vi "OPC UA Client-Read Historical Data.vi"() -> ()   [LabVIEW 2017]
uses:
  <vilib>/OPCUA/controls/History Data.ctl
  <vilib>/OPCUA/controls/OPC UA StatusCode.ctl
  <vilib>/OPCUA/NI OPC UA Client.lvlib
panel:
  out "XY Graph":cluster{"timestamp":timestamp, dbl}[](graph)=[{"timestamp"=timestamp(3600854440.93791 s since 1904-01-01), 21.20588510972274}, {"timestamp"=timestamp(3600854441.939849 s since 1904-01-01), 27.333235009001452}, {"timestamp"=timestamp(3600854442.9396653 s since 1904-01-01), 21.855502801352223}, {"timestamp"=timestamp(3600854443.9388895 s since 1904-01-01), 29.615495560358447}, {"timestamp"=timestamp(3600854444.939037 s since 1904-01-01), 22.706889869768354}, {"timestamp"=timestamp(3600854445.940808 s since 1904-01-01), 26.35983058252613}, {"timestamp"=timestamp(3600854446.941717 s since 1904-01-01), 21.221547649340067}, {"timestamp"=timestamp(3600854447.9409194 s since 1904-01-01), 27.220020293274708}, {"timestamp"=timestamp(3600854448.94098 s since 1904-01-01), 24.57336899433289}, {"timestamp"=timestamp(3600854449.941644 s since 1904-01-01), 28.626733755791868}, {"timestamp"=timestamp(3600854450.9408674 s since 1904-01-01), 20.70668111314054}, {"timestamp"=timestamp(3600854451.9410872 s since 1904-01-01), 26.09530969102767}, {"timestamp"=timestamp(3600854452.941859 s since 1904-01-01), 29.261574143396878}, {"timestamp"=timestamp(3600854453.94282 s since 1904-01-01), 22.263766443084574}, {"timestamp"=timestamp(3600854454.9423304 s since 1904-01-01), 29.772704225559018}, {"timestamp"=timestamp(3600854455.9420905 s since 1904-01-01), 22.457297555978183}, {"timestamp"=timestamp(3600854456.942924 s since 1904-01-01), 22.19965232198119}, {"timestamp"=timestamp(3600854457.9447994 s since 1904-01-01), 21.401399761563994}, {"timestamp"=timestamp(3600854458.9439445 s since 1904-01-01), 27.088882002360943}, {"timestamp"=timestamp(3600854459.943992 s since 1904-01-01), 22.602582119449764}, {"timestamp"=timestamp(3600854460.9440994 s since 1904-01-01), 29.08142660378008}, {"timestamp"=timestamp(3600854461.9441566 s since 1904-01-01), 28.630250179567135}, {"timestamp"=timestamp(3600854462.944467 s since 1904-01-01), 21.114338923136728}, {"timestamp"=timestamp(3600854463.944479 s since 1904-01-01), 25.125580129796955}, {"timestamp"=timestamp(3600854464.9440813 s since 1904-01-01), 23.49143403146742}, {"timestamp"=timestamp(3600854465.9448175 s since 1904-01-01), 24.15475262716179}, {"timestamp"=timestamp(3600854466.944839 s since 1904-01-01), 21.48417929583267}, {"timestamp"=timestamp(3600854467.9439993 s since 1904-01-01), 27.988717224834083}, {"timestamp"=timestamp(3600854468.9438586 s since 1904-01-01), 22.36166135322488}, {"timestamp"=timestamp(3600854469.943939 s since 1904-01-01), 21.126212489266607}, {"timestamp"=timestamp(3600854470.944815 s since 1904-01-01), 23.762638809610447}, {"timestamp"=timestamp(3600854471.9439936 s since 1904-01-01), 27.854304406099796}, {"timestamp"=timestamp(3600854472.9442863 s since 1904-01-01), 20.55133627589681}, {"timestamp"=timestamp(3600854473.944202 s since 1904-01-01), 22.098002254044697}, {"timestamp"=timestamp(3600854474.9439692 s since 1904-01-01), 28.157037330075237}, {"timestamp"=timestamp(3600854475.944336 s since 1904-01-01), 27.039356091430307}, {"timestamp"=timestamp(3600854476.9447656 s since 1904-01-01), 24.751319694406348}, {"timestamp"=timestamp(3600854477.9448185 s since 1904-01-01), 23.963820168468438}, {"timestamp"=timestamp(3600854478.944527 s since 1904-01-01), 20.20490890233939}, {"timestamp"=timestamp(3600854479.944155 s since 1904-01-01), 29.410268009654118}, {"timestamp"=timestamp(3600854480.943865 s since 1904-01-01), 21.843906881862438}, {"timestamp"=timestamp(3600854481.9445095 s since 1904-01-01), 21.10194055370115}, {"timestamp"=timestamp(3600854482.9444065 s since 1904-01-01), 20.555004281742956}, {"timestamp"=timestamp(3600854483.944839 s since 1904-01-01), 28.453532206994506}, {"timestamp"=timestamp(3600854484.9440255 s since 1904-01-01), 27.422547045358044}, {"timestamp"=timestamp(3600854485.9439983 s since 1904-01-01), 20.623258344377025}, {"timestamp"=timestamp(3600854486.944007 s since 1904-01-01), 28.23587856600172}, {"timestamp"=timestamp(3600854487.9439974 s since 1904-01-01), 23.665890936914323}, {"timestamp"=timestamp(3600854488.943952 s since 1904-01-01), 29.514702727179603}, {"timestamp"=timestamp(3600854489.944659 s since 1904-01-01), 24.022882267529802}, {"timestamp"=timestamp(3600854490.9439135 s since 1904-01-01), 26.30617869644069}, {"timestamp"=timestamp(3600854491.944177 s since 1904-01-01), 24.015406120491846}, {"timestamp"=timestamp(3600854492.944041 s since 1904-01-01), 21.548670361487137}, {"timestamp"=timestamp(3600854493.9443345 s since 1904-01-01), 20.7415449546357}, {"timestamp"=timestamp(3600854494.943878 s since 1904-01-01), 29.169815398048655}, {"timestamp"=timestamp(3600854495.9447403 s since 1904-01-01), 28.06303879063331}, {"timestamp"=timestamp(3600854496.944 s since 1904-01-01), 26.227528626788384}, {"timestamp"=timestamp(3600854497.944789 s since 1904-01-01), 22.616252795320047}, {"timestamp"=timestamp(3600854498.9439983 s since 1904-01-01), 27.346203051188446}, {"timestamp"=timestamp(3600854499.9446516 s since 1904-01-01), 27.909541180535452}, {"timestamp"=timestamp(3600854500.944337 s since 1904-01-01), 22.597281311339717}, {"timestamp"=timestamp(3600854501.9440007 s since 1904-01-01), 20.73793804733719}, {"timestamp"=timestamp(3600854502.944362 s since 1904-01-01), 22.135349424718896}, {"timestamp"=timestamp(3600854503.9450603 s since 1904-01-01), 22.480817410347225}, {"timestamp"=timestamp(3600854504.945788 s since 1904-01-01), 25.291304165035292}, {"timestamp"=timestamp(3600854505.945462 s since 1904-01-01), 24.71173765632412}, {"timestamp"=timestamp(3600854506.945313 s since 1904-01-01), 29.621885014310337}, {"timestamp"=timestamp(3600854507.945216 s since 1904-01-01), 25.453667341959644}, {"timestamp"=timestamp(3600854508.945589 s since 1904-01-01), 23.48524795814973}, {"timestamp"=timestamp(3600854509.9449096 s since 1904-01-01), 21.272583403623567}, {"timestamp"=timestamp(3600854510.944916 s since 1904-01-01), 24.770393157923007}, {"timestamp"=timestamp(3600854511.946425 s since 1904-01-01), 22.851024323085905}, {"timestamp"=timestamp(3600854512.9476576 s since 1904-01-01), 22.068332394286053}, {"timestamp"=timestamp(3600854513.947581 s since 1904-01-01), 20.10418987540174}, {"timestamp"=timestamp(3600854514.947266 s since 1904-01-01), 20.851516959644574}, {"timestamp"=timestamp(3600854515.946886 s since 1904-01-01), 21.788676349943273}, {"timestamp"=timestamp(3600854516.9470286 s since 1904-01-01), 24.364837290235858}, {"timestamp"=timestamp(3600854517.9473186 s since 1904-01-01), 21.753661420843862}, {"timestamp"=timestamp(3600854518.9468846 s since 1904-01-01), 20.668305189173065}, {"timestamp"=timestamp(3600854519.9477754 s since 1904-01-01), 29.19807367732829}, {"timestamp"=timestamp(3600854520.9470224 s since 1904-01-01), 20.794667983413667}, {"timestamp"=timestamp(3600854521.9469614 s since 1904-01-01), 26.923625793444977}, {"timestamp"=timestamp(3600854522.948755 s since 1904-01-01), 28.26477955665425}, {"timestamp"=timestamp(3600854523.9480367 s since 1904-01-01), 27.233847669422364}, {"timestamp"=timestamp(3600854524.9483833 s since 1904-01-01), 23.88384219554672}, {"timestamp"=timestamp(3600854525.948157 s since 1904-01-01), 23.200242776951892}, {"timestamp"=timestamp(3600854526.947979 s since 1904-01-01), 21.020485425211124}, {"timestamp"=timestamp(3600854527.948843 s since 1904-01-01), 28.14356476706218}, {"timestamp"=timestamp(3600854528.9480033 s since 1904-01-01), 20.520725665777498}, {"timestamp"=timestamp(3600854529.9478817 s since 1904-01-01), 25.289242939012087}, {"timestamp"=timestamp(3600854530.9488854 s since 1904-01-01), 23.86267595342772}, {"timestamp"=timestamp(3600854531.9489193 s since 1904-01-01), 27.741582204726043}, {"timestamp"=timestamp(3600854532.9495764 s since 1904-01-01), 26.03646242440425}, {"timestamp"=timestamp(3600854533.9489527 s since 1904-01-01), 23.905237458073483}, {"timestamp"=timestamp(3600854534.9501815 s since 1904-01-01), 23.516940804124538}, {"timestamp"=timestamp(3600854535.9502096 s since 1904-01-01), 22.530853600405738}, {"timestamp"=timestamp(3600854536.9508224 s since 1904-01-01), 28.7465433400168}, {"timestamp"=timestamp(3600854537.951188 s since 1904-01-01), 20.13545348870363}, {"timestamp"=timestamp(3600854538.9510765 s since 1904-01-01), 24.448939440228617}, {"timestamp"=timestamp(3600854539.9510746 s since 1904-01-01), 26.616814362460815}, {"timestamp"=timestamp(3600854540.9511366 s since 1904-01-01), 27.421849897221783}, {"timestamp"=timestamp(3600854541.9512854 s since 1904-01-01), 22.378214176762448}, {"timestamp"=timestamp(3600854542.952792 s since 1904-01-01), 26.992067160366545}, {"timestamp"=timestamp(3600854543.95334 s since 1904-01-01), 21.586544113894956}, {"timestamp"=timestamp(3600854544.953058 s since 1904-01-01), 21.7940680737806}, {"timestamp"=timestamp(3600854545.952887 s since 1904-01-01), 21.0186819021422}, {"timestamp"=timestamp(3600854546.953266 s since 1904-01-01), 27.3754869624632}, {"timestamp"=timestamp(3600854547.953187 s since 1904-01-01), 24.9426179621835}, {"timestamp"=timestamp(3600854548.95312 s since 1904-01-01), 23.35368046839681}, {"timestamp"=timestamp(3600854549.953189 s since 1904-01-01), 23.93699611757005}, {"timestamp"=timestamp(3600854550.9533286 s since 1904-01-01), 25.636595606336677}, {"timestamp"=timestamp(3600854551.9538 s since 1904-01-01), 26.889323355397032}, {"timestamp"=timestamp(3600854552.953631 s since 1904-01-01), 28.85079720214801}, {"timestamp"=timestamp(3600854553.954448 s since 1904-01-01), 28.731090207528318}, {"timestamp"=timestamp(3600854554.9552226 s since 1904-01-01), 21.767028993061967}, {"timestamp"=timestamp(3600854555.9550023 s since 1904-01-01), 27.833316777981892}, {"timestamp"=timestamp(3600854556.955756 s since 1904-01-01), 21.455427612682307}, {"timestamp"=timestamp(3600854557.9566555 s since 1904-01-01), 28.066436740378286}, {"timestamp"=timestamp(3600854558.957946 s since 1904-01-01), 22.283588668144777}, {"timestamp"=timestamp(3600854559.958628 s since 1904-01-01), 23.797763321462522}]
  out "history data":T1[](array[typedef])=[{"value "=variant(dbl 21.20588510972274), "timestamp"=timestamp(3600854440.93791 s since 1904-01-01), "node status"=0}, {"value "=variant(dbl 27.333235009001452), "timestamp"=timestamp(3600854441.939849 s since 1904-01-01), "node status"=0}, {"value "=variant(dbl 21.855502801352223), "timestamp"=timestamp(3600854442.9396653 s since 1904-01-01), "node status"=0}, {"value "=variant(dbl 29.615495560358447), "timestamp"=timestamp(3600854443.9388895 s since 1904-01-01), "node status"=0}, {"value "=variant(dbl 22.706889869768354), "timestamp"=timestamp(3600854444.939037 s since 1904-01-01), "node status"=0}, {"value "=variant(dbl 26.35983058252613), "timestamp"=timestamp(3600854445.940808 s since 1904-01-01), "node status"=0}, {"value "=variant(dbl 21.221547649340067), "timestamp"=timestamp(3600854446.941717 s since 1904-01-01), "node status"=0}, {"value "=variant(dbl 27.220020293274708), "timestamp"=timestamp(3600854447.9409194 s since 1904-01-01), "node status"=0}, {"value "=variant(dbl 24.57336899433289), "timestamp"=timestamp(3600854448.94098 s since 1904-01-01), "node status"=0}, {"value "=variant(dbl 28.626733755791868), "timestamp"=timestamp(3600854449.941644 s since 1904-01-01), "node status"=0}, {"value "=variant(dbl 20.70668111314054), "timestamp"=timestamp(3600854450.9408674 s since 1904-01-01), "node status"=0}, {"value "=variant(dbl 26.09530969102767), "timestamp"=timestamp(3600854451.9410872 s since 1904-01-01), "node status"=0}, {"value "=variant(dbl 29.261574143396878), "timestamp"=timestamp(3600854452.941859 s since 1904-01-01), "node status"=0}, {"value "=variant(dbl 22.263766443084574), "timestamp"=timestamp(3600854453.94282 s since 1904-01-01), "node status"=0}, {"value "=variant(dbl 29.772704225559018), "timestamp"=timestamp(3600854454.9423304 s since 1904-01-01), "node status"=0}, {"value "=variant(dbl 22.457297555978183), "timestamp"=timestamp(3600854455.9420905 s since 1904-01-01), "node status"=0}, {"value "=variant(dbl 22.19965232198119), "timestamp"=timestamp(3600854456.942924 s since 1904-01-01), "node status"=0}, {"value "=variant(dbl 21.401399761563994), "timestamp"=timestamp(3600854457.9447994 s since 1904-01-01), "node status"=0}, {"value "=variant(dbl 27.088882002360943), "timestamp"=timestamp(3600854458.9439445 s since 1904-01-01), "node status"=0}, {"value "=variant(dbl 22.602582119449764), "timestamp"=timestamp(3600854459.943992 s since 1904-01-01), "node status"=0}, {"value "=variant(dbl 29.08142660378008), "timestamp"=timestamp(3600854460.9440994 s since 1904-01-01), "node status"=0}, {"value "=variant(dbl 28.630250179567135), "timestamp"=timestamp(3600854461.9441566 s since 1904-01-01), "node status"=0}, {"value "=variant(dbl 21.114338923136728), "timestamp"=timestamp(3600854462.944467 s since 1904-01-01), "node status"=0}, {"value "=variant(dbl 25.125580129796955), "timestamp"=timestamp(3600854463.944479 s since 1904-01-01), "node status"=0}, {"value "=variant(dbl 23.49143403146742), "timestamp"=timestamp(3600854464.9440813 s since 1904-01-01), "node status"=0}, {"value "=variant(dbl 24.15475262716179), "timestamp"=timestamp(3600854465.9448175 s since 1904-01-01), "node status"=0}, {"value "=variant(dbl 21.48417929583267), "timestamp"=timestamp(3600854466.944839 s since 1904-01-01), "node status"=0}, {"value "=variant(dbl 27.988717224834083), "timestamp"=timestamp(3600854467.9439993 s since 1904-01-01), "node status"=0}, {"value "=variant(dbl 22.36166135322488), "timestamp"=timestamp(3600854468.9438586 s since 1904-01-01), "node status"=0}, {"value "=variant(dbl 21.126212489266607), "timestamp"=timestamp(3600854469.943939 s since 1904-01-01), "node status"=0}, {"value "=variant(dbl 23.762638809610447), "timestamp"=timestamp(3600854470.944815 s since 1904-01-01), "node status"=0}, {"value "=variant(dbl 27.854304406099796), "timestamp"=timestamp(3600854471.9439936 s since 1904-01-01), "node status"=0}, {"value "=variant(dbl 20.55133627589681), "timestamp"=timestamp(3600854472.9442863 s since 1904-01-01), "node status"=0}, {"value "=variant(dbl 22.098002254044697), "timestamp"=timestamp(3600854473.944202 s since 1904-01-01), "node status"=0}, {"value "=variant(dbl 28.157037330075237), "timestamp"=timestamp(3600854474.9439692 s since 1904-01-01), "node status"=0}, {"value "=variant(dbl 27.039356091430307), "timestamp"=timestamp(3600854475.944336 s since 1904-01-01), "node status"=0}, {"value "=variant(dbl 24.751319694406348), "timestamp"=timestamp(3600854476.9447656 s since 1904-01-01), "node status"=0}, {"value "=variant(dbl 23.963820168468438), "timestamp"=timestamp(3600854477.9448185 s since 1904-01-01), "node status"=0}, {"value "=variant(dbl 20.20490890233939), "timestamp"=timestamp(3600854478.944527 s since 1904-01-01), "node status"=0}, {"value "=variant(dbl 29.410268009654118), "timestamp"=timestamp(3600854479.944155 s since 1904-01-01), "node status"=0}, {"value "=variant(dbl 21.843906881862438), "timestamp"=timestamp(3600854480.943865 s since 1904-01-01), "node status"=0}, {"value "=variant(dbl 21.10194055370115), "timestamp"=timestamp(3600854481.9445095 s since 1904-01-01), "node status"=0}, {"value "=variant(dbl 20.555004281742956), "timestamp"=timestamp(3600854482.9444065 s since 1904-01-01), "node status"=0}, {"value "=variant(dbl 28.453532206994506), "timestamp"=timestamp(3600854483.944839 s since 1904-01-01), "node status"=0}, {"value "=variant(dbl 27.422547045358044), "timestamp"=timestamp(3600854484.9440255 s since 1904-01-01), "node status"=0}, {"value "=variant(dbl 20.623258344377025), "timestamp"=timestamp(3600854485.9439983 s since 1904-01-01), "node status"=0}, {"value "=variant(dbl 28.23587856600172), "timestamp"=timestamp(3600854486.944007 s since 1904-01-01), "node status"=0}, {"value "=variant(dbl 23.665890936914323), "timestamp"=timestamp(3600854487.9439974 s since 1904-01-01), "node status"=0}, {"value "=variant(dbl 29.514702727179603), "timestamp"=timestamp(3600854488.943952 s since 1904-01-01), "node status"=0}, {"value "=variant(dbl 24.022882267529802), "timestamp"=timestamp(3600854489.944659 s since 1904-01-01), "node status"=0}, {"value "=variant(dbl 26.30617869644069), "timestamp"=timestamp(3600854490.9439135 s since 1904-01-01), "node status"=0}, {"value "=variant(dbl 24.015406120491846), "timestamp"=timestamp(3600854491.944177 s since 1904-01-01), "node status"=0}, {"value "=variant(dbl 21.548670361487137), "timestamp"=timestamp(3600854492.944041 s since 1904-01-01), "node status"=0}, {"value "=variant(dbl 20.7415449546357), "timestamp"=timestamp(3600854493.9443345 s since 1904-01-01), "node status"=0}, {"value "=variant(dbl 29.169815398048655), "timestamp"=timestamp(3600854494.943878 s since 1904-01-01), "node status"=0}, {"value "=variant(dbl 28.06303879063331), "timestamp"=timestamp(3600854495.9447403 s since 1904-01-01), "node status"=0}, {"value "=variant(dbl 26.227528626788384), "timestamp"=timestamp(3600854496.944 s since 1904-01-01), "node status"=0}, {"value "=variant(dbl 22.616252795320047), "timestamp"=timestamp(3600854497.944789 s since 1904-01-01), "node status"=0}, {"value "=variant(dbl 27.346203051188446), "timestamp"=timestamp(3600854498.9439983 s since 1904-01-01), "node status"=0}, {"value "=variant(dbl 27.909541180535452), "timestamp"=timestamp(3600854499.9446516 s since 1904-01-01), "node status"=0}, {"value "=variant(dbl 22.597281311339717), "timestamp"=timestamp(3600854500.944337 s since 1904-01-01), "node status"=0}, {"value "=variant(dbl 20.73793804733719), "timestamp"=timestamp(3600854501.9440007 s since 1904-01-01), "node status"=0}, {"value "=variant(dbl 22.135349424718896), "timestamp"=timestamp(3600854502.944362 s since 1904-01-01), "node status"=0}, {"value "=variant(dbl 22.480817410347225), "timestamp"=timestamp(3600854503.9450603 s since 1904-01-01), "node status"=0}, {"value "=variant(dbl 25.291304165035292), "timestamp"=timestamp(3600854504.945788 s since 1904-01-01), "node status"=0}, {"value "=variant(dbl 24.71173765632412), "timestamp"=timestamp(3600854505.945462 s since 1904-01-01), "node status"=0}, {"value "=variant(dbl 29.621885014310337), "timestamp"=timestamp(3600854506.945313 s since 1904-01-01), "node status"=0}, {"value "=variant(dbl 25.453667341959644), "timestamp"=timestamp(3600854507.945216 s since 1904-01-01), "node status"=0}, {"value "=variant(dbl 23.48524795814973), "timestamp"=timestamp(3600854508.945589 s since 1904-01-01), "node status"=0}, {"value "=variant(dbl 21.272583403623567), "timestamp"=timestamp(3600854509.9449096 s since 1904-01-01), "node status"=0}, {"value "=variant(dbl 24.770393157923007), "timestamp"=timestamp(3600854510.944916 s since 1904-01-01), "node status"=0}, {"value "=variant(dbl 22.851024323085905), "timestamp"=timestamp(3600854511.946425 s since 1904-01-01), "node status"=0}, {"value "=variant(dbl 22.068332394286053), "timestamp"=timestamp(3600854512.9476576 s since 1904-01-01), "node status"=0}, {"value "=variant(dbl 20.10418987540174), "timestamp"=timestamp(3600854513.947581 s since 1904-01-01), "node status"=0}, {"value "=variant(dbl 20.851516959644574), "timestamp"=timestamp(3600854514.947266 s since 1904-01-01), "node status"=0}, {"value "=variant(dbl 21.788676349943273), "timestamp"=timestamp(3600854515.946886 s since 1904-01-01), "node status"=0}, {"value "=variant(dbl 24.364837290235858), "timestamp"=timestamp(3600854516.9470286 s since 1904-01-01), "node status"=0}, {"value "=variant(dbl 21.753661420843862), "timestamp"=timestamp(3600854517.9473186 s since 1904-01-01), "node status"=0}, {"value "=variant(dbl 20.668305189173065), "timestamp"=timestamp(3600854518.9468846 s since 1904-01-01), "node status"=0}, {"value "=variant(dbl 29.19807367732829), "timestamp"=timestamp(3600854519.9477754 s since 1904-01-01), "node status"=0}, {"value "=variant(dbl 20.794667983413667), "timestamp"=timestamp(3600854520.9470224 s since 1904-01-01), "node status"=0}, {"value "=variant(dbl 26.923625793444977), "timestamp"=timestamp(3600854521.9469614 s since 1904-01-01), "node status"=0}, {"value "=variant(dbl 28.26477955665425), "timestamp"=timestamp(3600854522.948755 s since 1904-01-01), "node status"=0}, {"value "=variant(dbl 27.233847669422364), "timestamp"=timestamp(3600854523.9480367 s since 1904-01-01), "node status"=0}, {"value "=variant(dbl 23.88384219554672), "timestamp"=timestamp(3600854524.9483833 s since 1904-01-01), "node status"=0}, {"value "=variant(dbl 23.200242776951892), "timestamp"=timestamp(3600854525.948157 s since 1904-01-01), "node status"=0}, {"value "=variant(dbl 21.020485425211124), "timestamp"=timestamp(3600854526.947979 s since 1904-01-01), "node status"=0}, {"value "=variant(dbl 28.14356476706218), "timestamp"=timestamp(3600854527.948843 s since 1904-01-01), "node status"=0}, {"value "=variant(dbl 20.520725665777498), "timestamp"=timestamp(3600854528.9480033 s since 1904-01-01), "node status"=0}, {"value "=variant(dbl 25.289242939012087), "timestamp"=timestamp(3600854529.9478817 s since 1904-01-01), "node status"=0}, {"value "=variant(dbl 23.86267595342772), "timestamp"=timestamp(3600854530.9488854 s since 1904-01-01), "node status"=0}, {"value "=variant(dbl 27.741582204726043), "timestamp"=timestamp(3600854531.9489193 s since 1904-01-01), "node status"=0}, {"value "=variant(dbl 26.03646242440425), "timestamp"=timestamp(3600854532.9495764 s since 1904-01-01), "node status"=0}, {"value "=variant(dbl 23.905237458073483), "timestamp"=timestamp(3600854533.9489527 s since 1904-01-01), "node status"=0}, {"value "=variant(dbl 23.516940804124538), "timestamp"=timestamp(3600854534.9501815 s since 1904-01-01), "node status"=0}, {"value "=variant(dbl 22.530853600405738), "timestamp"=timestamp(3600854535.9502096 s since 1904-01-01), "node status"=0}, {"value "=variant(dbl 28.7465433400168), "timestamp"=timestamp(3600854536.9508224 s since 1904-01-01), "node status"=0}, {"value "=variant(dbl 20.13545348870363), "timestamp"=timestamp(3600854537.951188 s since 1904-01-01), "node status"=0}, {"value "=variant(dbl 24.448939440228617), "timestamp"=timestamp(3600854538.9510765 s since 1904-01-01), "node status"=0}, {"value "=variant(dbl 26.616814362460815), "timestamp"=timestamp(3600854539.9510746 s since 1904-01-01), "node status"=0}, {"value "=variant(dbl 27.421849897221783), "timestamp"=timestamp(3600854540.9511366 s since 1904-01-01), "node status"=0}, {"value "=variant(dbl 22.378214176762448), "timestamp"=timestamp(3600854541.9512854 s since 1904-01-01), "node status"=0}, {"value "=variant(dbl 26.992067160366545), "timestamp"=timestamp(3600854542.952792 s since 1904-01-01), "node status"=0}, {"value "=variant(dbl 21.586544113894956), "timestamp"=timestamp(3600854543.95334 s since 1904-01-01), "node status"=0}, {"value "=variant(dbl 21.7940680737806), "timestamp"=timestamp(3600854544.953058 s since 1904-01-01), "node status"=0}, {"value "=variant(dbl 21.0186819021422), "timestamp"=timestamp(3600854545.952887 s since 1904-01-01), "node status"=0}, {"value "=variant(dbl 27.3754869624632), "timestamp"=timestamp(3600854546.953266 s since 1904-01-01), "node status"=0}, {"value "=variant(dbl 24.9426179621835), "timestamp"=timestamp(3600854547.953187 s since 1904-01-01), "node status"=0}, {"value "=variant(dbl 23.35368046839681), "timestamp"=timestamp(3600854548.95312 s since 1904-01-01), "node status"=0}, {"value "=variant(dbl 23.93699611757005), "timestamp"=timestamp(3600854549.953189 s since 1904-01-01), "node status"=0}, {"value "=variant(dbl 25.636595606336677), "timestamp"=timestamp(3600854550.9533286 s since 1904-01-01), "node status"=0}, {"value "=variant(dbl 26.889323355397032), "timestamp"=timestamp(3600854551.9538 s since 1904-01-01), "node status"=0}, {"value "=variant(dbl 28.85079720214801), "timestamp"=timestamp(3600854552.953631 s since 1904-01-01), "node status"=0}, {"value "=variant(dbl 28.731090207528318), "timestamp"=timestamp(3600854553.954448 s since 1904-01-01), "node status"=0}, {"value "=variant(dbl 21.767028993061967), "timestamp"=timestamp(3600854554.9552226 s since 1904-01-01), "node status"=0}, {"value "=variant(dbl 27.833316777981892), "timestamp"=timestamp(3600854555.9550023 s since 1904-01-01), "node status"=0}, {"value "=variant(dbl 21.455427612682307), "timestamp"=timestamp(3600854556.955756 s since 1904-01-01), "node status"=0}, {"value "=variant(dbl 28.066436740378286), "timestamp"=timestamp(3600854557.9566555 s since 1904-01-01), "node status"=0}, {"value "=variant(dbl 22.283588668144777), "timestamp"=timestamp(3600854558.957946 s since 1904-01-01), "node status"=0}, {"value "=variant(dbl 23.797763321462522), "timestamp"=timestamp(3600854559.958628 s since 1904-01-01), "node status"=0}] {"node status" items=["Good"=0, "Good_SubscriptionTransferred"=2949120, "Good_CompletesAsynchronously"=3014656, "Good_Overload"=3080192, "Good_Clamped"=3145728, "Good_LocalOverride"=9830400, "Good_EntryInserted"=10616832, "Good_EntryReplaced"=10682368, "Good_NoData"=10813440, "Good_MoreData"=10878976, "Good_CommunicationEvent"=10944512, "Good_ShutdownEvent"=11010048, "Good_CallAgain"=11075584, "Good_NonCriticalTimeout"=11141120, "Good_ResultsMayBeIncomplete"=12189696, "Good_DataIgnored"=14221312, "Uncertain_ReferenceOutOfServer"=1080819712, "Uncertain_NoCommunicationLastUsableValue"=1083113472, "Uncertain_LastUsableValue"=1083179008, "Uncertain_SubstituteValue"=1083244544, "Uncertain_InitialValue"=1083310080, "Uncertain_SensorNotAccurate"=1083375616, "Uncertain_EngineeringUnitsExceeded"=1083441152, "Uncertain_SubNormal"=1083506688, "Uncertain_DataSubNormal"=1084489728, "Uncertain_ReferenceNotDeleted"=1086062592, "Uncertain_NotAllNodesAvailable"=1086324736, "Bad_UnexpectedError"=2147549184, "Bad_InternalError"=2147614720, "Bad_OutOfMemory"=2147680256, "Bad_ResourceUnavailable"=2147745792, "Bad_CommunicationError"=2147811328, "Bad_EncodingError"=2147876864, "Bad_DecodingError"=2147942400, "Bad_EncodingLimitsExceeded"=2148007936, "Bad_UnknownResponse"=2148073472, "Bad_Timeout"=2148139008, "Bad_ServiceUnsupported"=2148204544, "Bad_Shutdown"=2148270080, "Bad_ServerNotConnected"=2148335616, "Bad_ServerHalted"=2148401152, "Bad_NothingToDo"=2148466688, "Bad_TooManyOperations"=2148532224, "Bad_DataTypeIdUnknown"=2148597760, "Bad_CertificateInvalid"=2148663296, "Bad_SecurityChecksFailed"=2148728832, "Bad_CertificateTimeInvalid"=2148794368, "Bad_CertificateIssuerTimeInvalid"=2148859904, "Bad_CertificateHostNameInvalid"=2148925440, "Bad_CertificateUriInvalid"=2148990976, "Bad_CertificateUseNotAllowed"=2149056512, "Bad_CertificateIssuerUseNotAllowed"=2149122048, "Bad_CertificateUntrusted"=2149187584, "Bad_CertificateRevocationUnknown"=2149253120, "Bad_CertificateIssuerRevocationUnknown"=2149318656, "Bad_CertificateRevoked"=2149384192, "Bad_CertificateIssuerRevoked"=2149449728, "Bad_UserAccessDenied"=2149515264, "Bad_IdentityTokenInvalid"=2149580800, "Bad_IdentityTokenRejected"=2149646336, "Bad_SecureChannelIdInvalid"=2149711872, "Bad_InvalidTimestamp"=2149777408, "Bad_NonceInvalid"=2149842944, "Bad_SessionIdInvalid"=2149908480, "Bad_SessionClosed"=2149974016, "Bad_SessionNotActivated"=2150039552, "Bad_SubscriptionIdInvalid"=2150105088, "Bad_RequestHeaderInvalid"=2150236160, "Bad_TimestampsToReturnInvalid"=2150301696, "Bad_RequestCancelledByClient"=2150367232, "Bad_NoCommunication"=2150694912, "Bad_WaitingForInitialData"=2150760448, "Bad_NodeIdInvalid"=2150825984, "Bad_NodeIdUnknown"=2150891520, "Bad_AttributeIdInvalid"=2150957056, "Bad_IndexRangeInvalid"=2151022592, "Bad_IndexRangeNoData"=2151088128, "Bad_DataEncodingInvalid"=2151153664, "Bad_DataEncodingUnsupported"=2151219200, "Bad_NotReadable"=2151284736, "Bad_NotWritable"=2151350272, "Bad_OutOfRange"=2151415808, "Bad_NotSupported"=2151481344, "Bad_NotFound"=2151546880, "Bad_ObjectDeleted"=2151612416, "Bad_NotImplemented"=2151677952, "Bad_MonitoringModeInvalid"=2151743488, "Bad_MonitoredItemIdInvalid"=2151809024, "Bad_MonitoredItemFilterInvalid"=2151874560, "Bad_MonitoredItemFilterUnsupported"=2151940096, "Bad_FilterNotAllowed"=2152005632, "Bad_StructureMissing"=2152071168, "Bad_EventFilterInvalid"=2152136704, "Bad_ContentFilterInvalid"=2152202240, "Bad_FilterOperandInvalid"=2152267776, "Bad_ContinuationPointInvalid"=2152333312, "Bad_NoContinuationPoints"=2152398848, "Bad_ReferenceTypeIdInvalid"=2152464384, "Bad_BrowseDirectionInvalid"=2152529920, "Bad_NodeNotInView"=2152595456, "Bad_ServerUriInvalid"=2152660992, "Bad_ServerNameMissing"=2152726528, "Bad_DiscoveryUrlMissing"=2152792064, "Bad_SempahoreFileMissing"=2152857600, "Bad_RequestTypeInvalid"=2152923136, "Bad_SecurityModeRejected"=2152988672, "Bad_SecurityPolicyRejected"=2153054208, "Bad_TooManySessions"=2153119744, "Bad_UserSignatureInvalid"=2153185280, "Bad_ApplicationSignatureInvalid"=2153250816, "Bad_NoValidCertificates"=2153316352, "Bad_RequestCancelledByRequest"=2153381888, "Bad_ParentNodeIdInvalid"=2153447424, "Bad_ReferenceNotAllowed"=2153512960, "Bad_NodeIdRejected"=2153578496, "Bad_NodeIdExists"=2153644032, "Bad_NodeClassInvalid"=2153709568, "Bad_BrowseNameInvalid"=2153775104, "Bad_BrowseNameDuplicated"=2153840640, "Bad_NodeAttributesInvalid"=2153906176, "Bad_TypeDefinitionInvalid"=2153971712, "Bad_SourceNodeIdInvalid"=2154037248, "Bad_TargetNodeIdInvalid"=2154102784, "Bad_DuplicateReferenceNotAllowed"=2154168320, "Bad_InvalidSelfReference"=2154233856, "Bad_ReferenceLocalOnly"=2154299392, "Bad_NoDeleteRights"=2154364928, "Bad_ServerIndexInvalid"=2154430464, "Bad_ViewIdUnknown"=2154496000, "Bad_TooManyMatches"=2154627072, "Bad_QueryTooComplex"=2154692608, "Bad_NoMatch"=2154758144, "Bad_MaxAgeInvalid"=2154823680, "Bad_HistoryOperationInvalid"=2154889216, "Bad_HistoryOperationUnsupported"=2154954752, "Bad_WriteNotSupported"=2155020288, "Bad_TypeMismatch"=2155085824, "Bad_MethodInvalid"=2155151360, "Bad_ArgumentsMissing"=2155216896, "Bad_TooManySubscriptions"=2155282432, "Bad_TooManyPublishRequests"=2155347968, "Bad_NoSubscription"=2155413504, "Bad_SequenceNumberUnknown"=2155479040, "Bad_MessageNotAvailable"=2155544576, "Bad_InsufficientClientProfile"=2155610112, "Bad_TcpServerTooBusy"=2155675648, "Bad_TcpMessageTypeInvalid"=2155741184, "Bad_TcpSecureChannelUnknown"=2155806720, "Bad_TcpMessageTooLarge"=2155872256, "Bad_TcpNotEnoughResources"=2155937792, "Bad_TcpInternalError"=2156003328, "Bad_TcpEndpointUrlInvalid"=2156068864, "Bad_RequestInterrupted"=2156134400, "Bad_RequestTimeout"=2156199936, "Bad_SecureChannelClosed"=2156265472, "Bad_SecureChannelTokenUnknown"=2156331008, "Bad_SequenceNumberInvalid"=2156396544, "Bad_ConfigurationError"=2156462080, "Bad_NotConnected"=2156527616, "Bad_DeviceFailure"=2156593152, "Bad_SensorFailure"=2156658688, "Bad_OutOfService"=2156724224, "Bad_DeadbandFilterInvalid"=2156789760, "Bad_RefreshInProgress"=2157379584, "Bad_ConditionAlreadyDisabled"=2157445120, "Bad_ConditionDisabled"=2157510656, "Bad_EventIdUnknown"=2157576192, "Bad_NoData"=2157641728, "Bad_DataLost"=2157772800, "Bad_DataUnavailable"=2157838336, "Bad_EntryExists"=2157903872, "Bad_NoEntryExists"=2157969408, "Bad_TimestampNotSupported"=2158034944, "Bad_InvalidArgument"=2158690304, "Bad_ConnectionRejected"=2158755840, "Bad_Disconnect"=2158821376, "Bad_ConnectionClosed"=2158886912, "Bad_InvalidState"=2158952448, "Bad_EndOfStream"=2159017984, "Bad_NoDataAvailable"=2159083520, "Bad_WaitingForResponse"=2159149056, "Bad_OperationAbandoned"=2159214592, "Bad_ExpectedStreamToBlock"=2159280128, "Bad_WouldBlock"=2159345664, "Bad_SyntaxError"=2159411200, "Bad_MaxConnectionsReached"=2159476736, "Bad_RequestTooLarge"=2159542272, "Bad_ResponseTooLarge"=2159607808, "Bad_EventNotAcknowledgeable"=2159738880, "Bad_InvalidTimestampArgument"=2159869952, "Bad_ProtocolVersionUnsupported"=2159935488, "Bad_StateNotActive"=2160001024, "Bad_FilterOperatorInvalid"=2160132096, "Bad_FilterOperatorUnsupported"=2160197632, "Bad_FilterOperandCountMismatch"=2160263168, "Bad_FilterElementInvalid"=2160328704, "Bad_FilterLiteralInvalid"=2160394240, "Bad_IdentityChangeNotSupported"=2160459776, "Bad_NotTypeDefinition"=2160590848, "Bad_ViewTimestampInvalid"=2160656384, "Bad_ViewParameterMismatch"=2160721920, "Bad_ViewVersionInvalid"=2160787456, "Bad_ConditionAlreadyEnabled"=2160852992, "Bad_DialogNotActive"=2160918528, "Bad_DialogResponseInvalid"=2160984064, "Bad_ConditionBranchAlreadyAcked"=2161049600, "Bad_ConditionBranchAlreadyConfirmed"=2161115136, "Bad_ConditionAlreadyShelved"=2161180672, "Bad_ConditionNotShelved"=2161246208, "Bad_ShelvingTimeOutOfRange"=2161311744, "Bad_AggregateListMismatch"=2161377280, "Bad_AggregateNotSupported"=2161442816, "Bad_AggregateInvalidInputs"=2161508352, "Bad_BoundNotFound"=2161573888, "Bad_BoundNotSupported"=2161639424, "Bad_AggregateConfigurationRejected"=2161770496, "Bad_TooManyMonitoredItems"=2161836032]}
  in  "request":T3={"start time"=timestamp(3600766624.048195 s since 1904-01-01), "end time"=timestamp(3600939412.567801 s since 1904-01-01), "num values per node"=0, "return bounds"=FALSE} {"start time" format="%<%H:%M:%S\n%Y/%m/%d>T"; "end time" format="%<%H:%M:%S\n%Y/%m/%d>T"}
  in  "Node Id":string="Process Data.Temperature"
  in  "Server Endpoint URL":string="opc.tcp://XPS15HPH:49580"
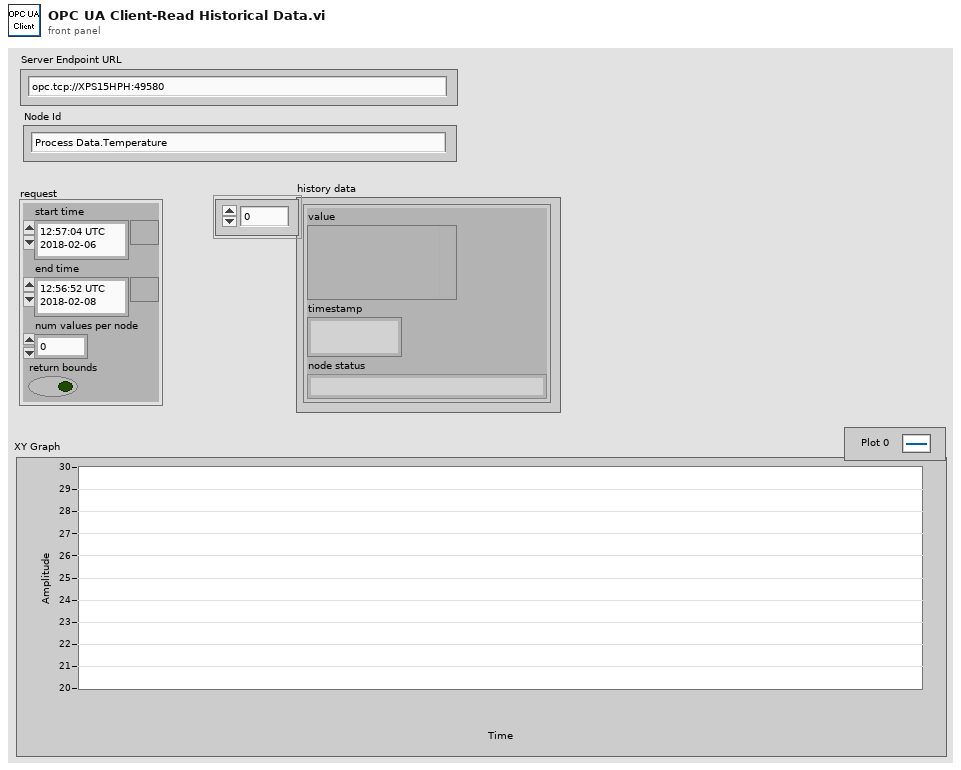
[diagram p1: front panel]
types:
  T1 = typedef "History Data.ctl" = cluster{"value ":variant, "timestamp":timestamp, "node status":T2}
  T2 = typedef "OPC UA StatusCode.ctl" = u32
  T3 = cluster{"start time":timestamp, "end time":timestamp, "num values per node":u32, "return bounds":bool}
  T4 = cluster{"message mode":enum16{"None", "Sign", "Sign and Encrypt"}, "security":enum16{"Basic256", "Basic128Rsa15"}}
  T5 = typedef "OPC UA Client Refnum.ctl" = refnum<k21>
  T6 = typedef "History Data Result.ctl" = cluster{"node ID":T7, "history data":T1[], "status":T2}
  T7 = typedef "NodeId.ctl" = string
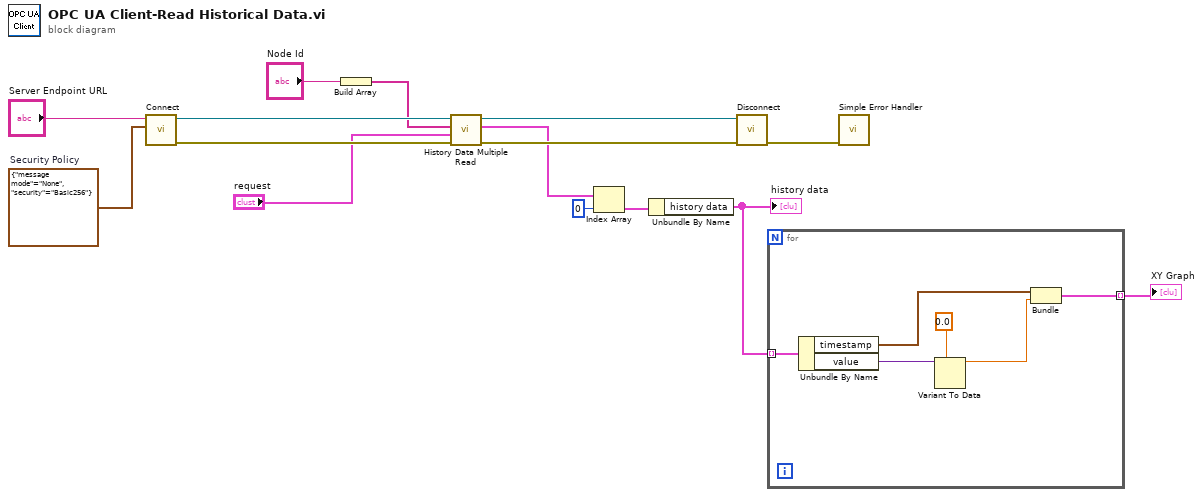
[diagram p0: block diagram]
diagram:
  w12 = T4 {"message mode"=enum."None", "security"=enum."Basic256"}  # Security Policy
  n1 = call <vilib>:"Connect.vi"("security policy"=w12, "server endpoint URL"="Server Endpoint URL") -> ("error out"=w8:errorcluster, "OPC UA client refnum out"=w15:T5)  [unwired: 7 in, 1 out]
  n2 = Build Array("Node Id") -> (w9:string[])
  n3 = call <vilib>:"History Data Multiple Read.vi"("error in (no error)"=w8, "request"="request", "node IDs"=w9, "OPC UA client refnum in"=w15) -> ("error out"=w7:errorcluster, "results"=w5:T6[], "OPC UA client refnum out"=w11:T5)  [unwired: 3 in, 2 out]
  n4 = Index Array(array=w5, index=0) -> (element=w3:T6)
  n5 = Unbundle By Name(w3) -> ("history data"=w2:T1[])
  "history data" <- w2
  n6 = call <vilib>:"Disconnect.vi"("error in (no error)"=w7, "OPC UA client refnum in"=w11) -> ("error out"=w14:errorcluster)  [unwired: 9 in]
  n7 = for {
    tunnel: w2 -> [w21] mode=indexing
    tunnel: [w16] -> w1 mode=indexing
    n8 = Unbundle By Name "Unbundle By Name"(w21) -> ("timestamp"=w18:timestamp, "value"=w20:variant)
    n9 = Variant To Data(type=0.0, Variant=w20) -> (data=w17:dbl)  [unwired: 1 in, 1 out]
    n10 = Bundle "Bundle"("timestamp"=w18, w17) -> (w16:cluster{"timestamp":timestamp, dbl})  [unwired: 1 in]
  }
  "XY Graph" <- w1
  n11 = call <vilib>:"Simple Error Handler.vi"("error in (no error)"=w14) -> ()  [unwired: 4 in, 5 out]
